vi "Move.vi"(8 "error in (no error)":errorcluster, 10 "target pos":dbl, 11 "VacuumLine in":refnum<class "VacuumLine.lvclass">) -> (0 "error out":errorcluster, 3 "VacuumLine out":refnum<class "VacuumLine.lvclass">)   [LabVIEW 2016, in "Hardware.lvlib" / "VacuumLine.lvlib" / "VacuumLine.lvclass"]
uses:
  <userlib>/Common Components/Hardware/Abstract System/VacuumLine/VacuumLine/VacuumLine.lvclass
  <userlib>/Common Components/Hardware/Abstract System/VacuumLine/VacuumLine/VacuumLine.lvclass/VacuumLine.ctl
  <userlib>/Common Components/Hardware/Motor/Motor/Motor.lvclass
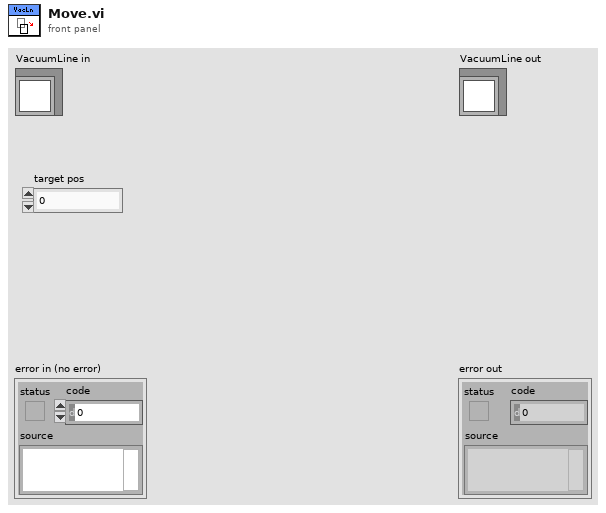
[diagram p1: front panel]
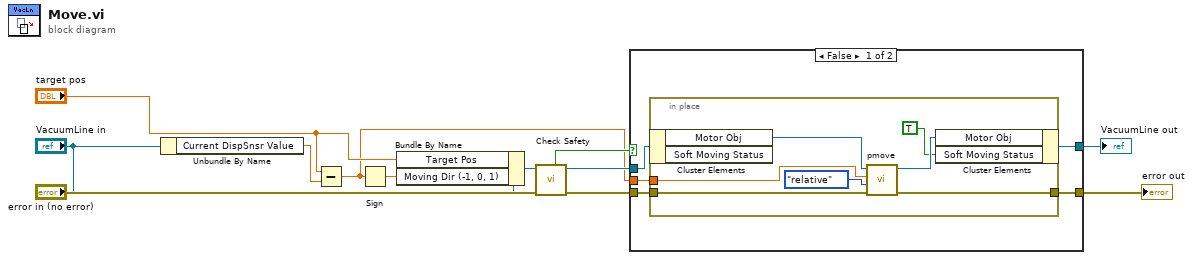
[diagram p0: block diagram]
diagram:
  n1 = Unbundle By Name("VacuumLine in") -> ("Current DispSnsr Value"=w5:dbl)
  n2 = Subtract(x="target pos", y=w5) -> (x-y=w1:dbl)
  n3 = Sign(1:w1) -> (0:w4:dbl)
  n4 = Bundle By Name(cluster="VacuumLine in", "Target Pos"="target pos", "Moving Dir (-1, 0, 1)"=w4) -> (w7:refnum<class "VacuumLine.lvclass">)
  n5 = call <userlib>:"Check Safety.vi"("error in (no error)"="error in (no error)", "VacuumLine in"=w7) -> ("error out"=w9:errorcluster, "VacuumLine out"=w8:refnum<class "VacuumLine.lvclass">, "Error"=w3:bool)  [unwired: 5 in, 2 out]
  n6 = case shown="False" w3 {
    tunnel: [w17 w25] -> w11
    tunnel: [w16 w26] -> w10
    tunnel: w9 -> [w15 w25]
    tunnel: w8 -> [w14 w26]
    tunnel: w1 -> [w13 _]
    frame False {
      n7 = in-place {
        in-place-border: w15 -> [w24]
        in-place-border: [w23] -> w17
        in-place-border: w13 -> [w21]
        n8 = in-place-cluster #1(w14) -> ("Motor Obj"=w19:refnum<class "Motor.lvclass">)  [unwired: 1 out]
        n9 = call <userlib>:"pmove.vi"("error in (no error)"=w24, "mode (0: rel; 1: abs)"=enum16{"relative", "absolute"}."relative", "distance in unit mode"=w21, "Motor in"=w19) -> ("error out"=w23:errorcluster, "Motor out"=w22:refnum<class "Motor.lvclass">)  [unwired: 6 in]
        n10 = in-place-cluster #1("Motor Obj"=w22, "Soft Moving Status"=TRUE) -> (w16:refnum<class "VacuumLine.lvclass">)
      }
    }
    frame True {
    }
  }
  "error out" <- w11
  "VacuumLine out" <- w10
